vi "IDS Make Even.vi"(7 "Input":i32) -> (8 "Even Output":i32)   [LabVIEW 2025]
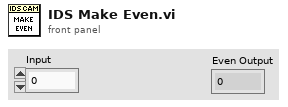
[diagram p1: front panel]
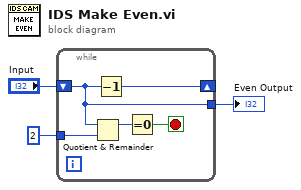
[diagram p0: block diagram]
diagram:
  n1 = while {
    shift-right: [w5] -> _
    shift-left: "Input" -> [w4]
    tunnel: 2 ("Allowed Increment") -> [w8]
    tunnel: [w4] -> w1
    stop <- w6 stop-if-true
    n2 = Quotient & Remainder(x=w4, y=w8) -> (x-y*floor(x/y)=w7:i32)  [unwired: 1 out]
    n3 = Decrement(x=w4) -> (x-1=w5:i32)
    n4 = Equal To 0?(x=w7) -> (x = 0?=w6:bool)
  }
  "Even Output" <- w1
